vi "DSF.Shared.Configuration.Framework.Cluster to Objects.vi"(8 "error in (no error)":errorcluster, 11 "Framework Configuration in":refnum<class "DSF.Shared.Configuration.Framework.lvclass">) -> (0 "error out":errorcluster, 3 "Framework Configuration out":refnum<class "DSF.Shared.Configuration.Framework.lvclass">)   [LabVIEW 2017, in "DSF.Shared.lvlib" / "DSF.Shared.Configuration.Framework.lvclass"]
uses:
  DSF.Shared.Configuration.Framework.lvclass
  DSF.Shared.Configuration.Framework.lvclass/DSF.Shared.Configuration.Framework.ctl
  Plugin/DSF.Shared.Configuration.Plugin.lvclass
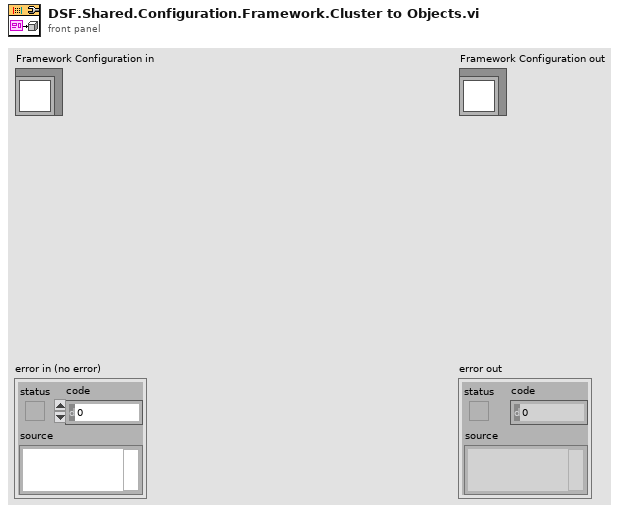
[diagram p1: front panel]
types:
  T1 = typedef "DSF.Shared.lvlib/DSF.Shared.Refactor.Typedefs.Framework Configuration.Aggregate.ctl" = cluster{"Plugins":T2[]}
  T2 = typedef "DSF.Shared.lvlib/DSF.Shared.Refactor.Typedefs.Plugin Configuration.Aggregate.ctl" = cluster{"name":string, "class":string, "cycle timing":T3, "Transfer Groups":T4[]}
  T3 = typedef "DSF.Shared.lvlib/DSF.Shared.Typedefs.Cycle Timing Factors.ctl" = cluster{"Priority":u64, "Decimation":u64, "Offset":u64}
  T4 = typedef "DSF.Shared.lvlib/DSF.Shared.Refactor.Typedefs.Transfer Group Configuration.Aggregate.ctl" = cluster{"name":string, "direction":T5, "cycle timing":T3, "Transfers":T6[]}
  T5 = typedef "DSF.Shared.lvlib/DSF.Shared.Typedefs.Direction.ctl" = enum8{"Tx", "Rx"}
  T6 = typedef "DSF.Shared.lvlib/DSF.Shared.Refactor.Typedefs.Transfer Configuration.ctl" = cluster{"name":string, "byte order":T7, "channel configurations":T8[]}
  T7 = typedef "DSF.Shared.lvlib/DSF.Shared.Typedefs.Byte Order.ctl" = enum8{"big-endian", "little-endian"}
  T8 = typedef "DSF.Shared.lvlib/DSF.Shared.Refactor.Typedefs.Channel Array Configuration.ctl" = cluster{"name":string, "data type":T9, "count":u64, "buffer offset":u64, "engine offset":u64}
  T9 = typedef "DSF.Shared.lvlib/DSF.Shared.Typedefs.Data Type.ctl" = enum8{"Bool", "SGL", "DBL", "I8", "I16", "I32", "I64", "U8", "U16", "U32", "U64"}
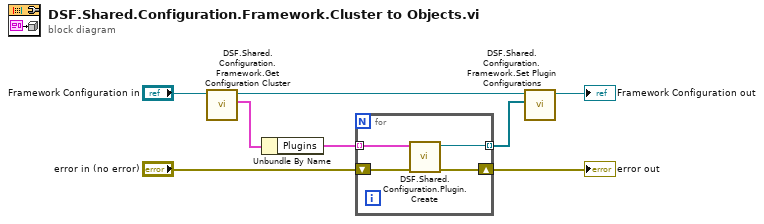
[diagram p0: block diagram]
diagram:
  n1 = call "DSF.Shared.Configuration.Framework.Get Configuration Cluster.vi"("Framework Configuration in"="Framework Configuration in") -> ("Framework Configuration"=w7:T1, "Framework Configuration out"=w3:refnum<class "DSF.Shared.Configuration.Framework.lvclass">)  [unwired: 9 in]
  n2 = Unbundle By Name(w7) -> ("Plugins"=w6:T2[])
  n3 = for {
    tunnel: w6 -> [w12] mode=indexing
    tunnel: [w11] -> w1 mode=indexing
    shift-right: [w10] -> w5
    shift-left: "error in (no error)" -> [w9]
    n4 = call "DSF.Shared.Configuration.Plugin.Create.vi"("error in (no error)"=w9, "Plugin Configuration cluster"=w12) -> ("error out"=w10:errorcluster, "Plugin Configuration"=w11:refnum<class "DSF.Shared.Configuration.Plugin.lvclass">)  [unwired: 8 in]
  }
  "error out" <- w5
  n5 = call "DSF.Shared.Configuration.Framework.Set Plugin Configurations.vi"("Plugin Configurations"=w1, "Framework Configuration in"=w3) -> ("Framework Configuration out"=→"Framework Configuration out":refnum<class "DSF.Shared.Configuration.Framework.lvclass">)  [unwired: 9 in]
